vi "8XY6.vi"(11 "Variables and Memory in":T1 {"GFX" format="%02x"}) -> (3 "Variables and Memory out":T1 {"GFX" format="%02x"})   [LabVIEW 2021]
uses:
  Controls/ClusterF.ctl
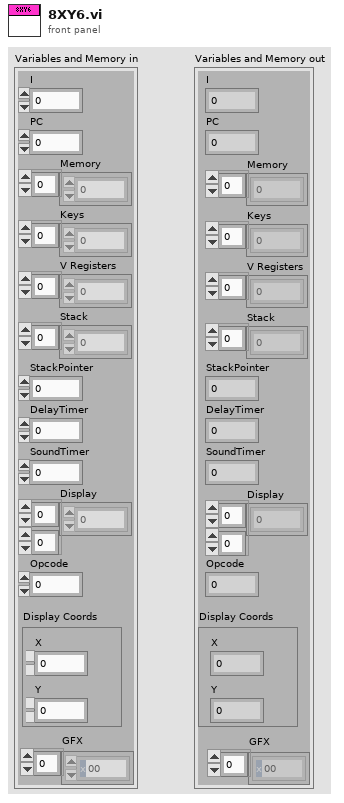
[diagram p1: front panel]
types:
  T1 = typedef "ClusterF.ctl" = cluster{"I":u16, "PC":u16, "Memory":u8[], "Keys":u8[], "V Registers":u8[], "Stack":u16[], "StackPointer":u16, "DelayTimer":u8, "SoundTimer":u8, "Display":u8[][], "Opcode":u16, "Display Coords":cluster{"X":u8, "Y":u8}, "GFX":u8[]}
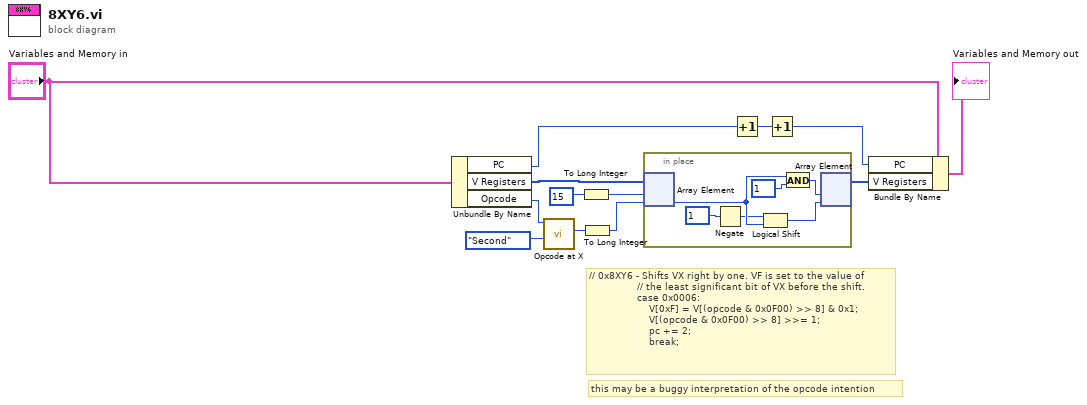
[diagram p0: block diagram]
diagram:
  # "this may be a buggy interpretation of the opcode intention"
  # "// 0x8XY6 - Shifts VX right by one. VF is set to the value of\n                // the least significant bit of VX before the shift.\n                case 0x0006:\n                    V[0xF] = V[(opcode & 0x0F00) >> 8] & 0x1;\n                    V[(opcode & 0x0F00) >> 8] >>= 1;\n                    pc += 2;\n                    break;"
  n1 = Unbundle By Name("Variables and Memory in") -> ("PC"=w12:u16, "V Registers"=w3:u8[], "Opcode"=w1:u16)
  n2 = call "Opcode at X.vi"("X Position"=enum16{"First", "Second", "Third", "Fourth"}."Second", "Opcode"=w1) -> ("Opcode at X Position (U8)"=w4:u8)  [unwired: 9 in]
  n3 = To Long Integer(number=u8 15 ("y")) -> (32bit integer=w7:i32)
  n4 = To Long Integer(number=w4) -> (32bit integer=w5:i32)
  n5 = in-place {
    n6 = in-place-array #1(w3, w7, w5) -> (w17:u8)  [unwired: 1 out]
    n7 = Negate(x=i8 1 ("y")) -> (-x=w16:i8)
    n8 = Logical Shift(y=w16, x=w17) -> (x << y=w14:u8)
    n9 = And(x=w17, y=u8 1) -> (x .and. y?=w18:u8)
    n10 = in-place-array #1(w18, w14) -> (w10:u8[])  [unwired: 2 out]
  }
  n11 = Increment(x=w12) -> (x+1=w11:u16)
  n12 = Increment(x=w11) -> (x+1=w13:u16)
  n13 = Bundle By Name(cluster="Variables and Memory in", "PC"=w13, "V Registers"=w10) -> (→"Variables and Memory out":T1)
